vi "Get Request Type.vi"(8 "error in (no error)":errorcluster, 11 "GetStats in":refnum<class "GetStats.lvclass">) -> (0 "error out":errorcluster, 2 "Request Type":string, 3 "GetStats out":refnum<class "GetStats.lvclass">)   [LabVIEW 2022 SP3, in "obs-websocket-lv.lvlib" / "GetStats.lvclass"]
uses:
  GetStats.lvclass
  GetStats.lvclass/GetStats.ctl
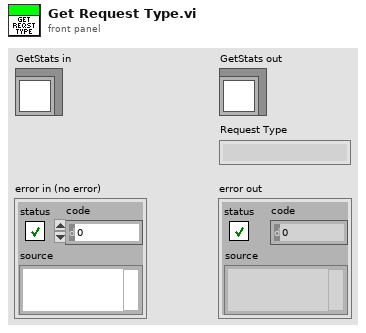
[diagram p1: front panel]
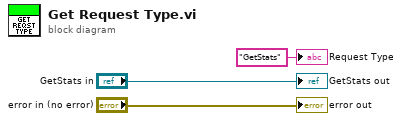
[diagram p0: block diagram]
diagram:
  "error out" <- "error in (no error)"
  "GetStats out" <- "GetStats in"
  "Request Type" <- "GetStats" ("Request Type")
